vi "Connect.vi"(8 "error in (no error)":errorcluster, 11 "DPO4104 in":refnum<class "DPO4104.lvclass">) -> (0 "error out":errorcluster, 3 "DPO4104 out":refnum<class "DPO4104.lvclass">)   [LabVIEW 2018, in "DPO4104.lvlib" / "DPO4104.lvclass"]
doc: "This Override method is used initiative the communication session with the Oscope instrument."
uses:
  DPO4104.lvclass
  PPLs/Oscilloscope/Parent/Oscilloscope.lvlibp/Oscilloscope.lvclass
  <instrlib>/Tektronix DPO MSO 2000 4000 Series/Tektronix DPO MSO 2000 4000 Series.lvlib
  C:/Projects/LabVIEW/PPLs/Oscilloscope/Parent/Oscilloscope.lvlibp/Oscilloscope.lvclass
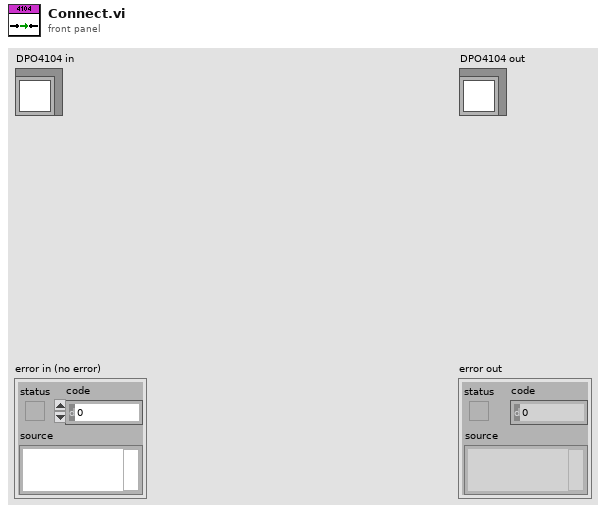
[diagram p1: front panel]
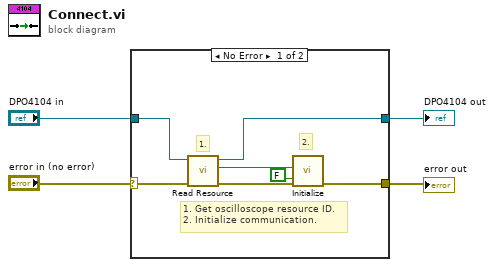
[diagram p0: block diagram]
diagram:
  n1 = case shown="No Error" "error in (no error)" {
    selector: "error in (no error)" -> [w11 w12]
    tunnel: [w9 w13] -> w2
    tunnel: "DPO4104 in" -> [w10 w13]
    tunnel: [w7 w12] -> w1
    frame No Error {
      # "2."
      # "1."
      # "1. Get oscilloscope resource ID.\n2. Initialize communication."
      n2 = call "Read Resource.vi"("error in (no error)"=w11, "Oscilloscope in"=w10) -> ("error out"=w8:errorcluster, "Resource"=w6:refnum<visa-resource-name>, "Oscilloscope out"=w9:refnum<class "DPO4104.lvclass">)  [unwired: 7 in]
      n3 = call <instrlib>:"Initialize.vi"("error in (no error)"=w8, "Reset (True)"=FALSE, "VISA resource name"=w6) -> ("error out"=w7:errorcluster)  [unwired: 7 in, 1 out]
    }
    frame Error {
    }
  }
  "error out" <- w1
  "DPO4104 out" <- w2
